vi "Thor_OpenDevice.vi"(8 "error in (no error)":errorcluster) -> (0 "error out":errorcluster, 2 "Device":T2, 3 "KCubeServoControl out":T1, 5 "CreateDevice?":bool)   [LabVIEW 2020]
uses:
  Thor_DeviceRef.ctl
  E:/Norway Project/All Hardware/New Microscope/LabVIEW/ThorLabs/ThorLabs.MotionControl.KCube.DCServoCLI.dll
  ThorLabs.MotionControl.KCube.DCServoCLI.dll
  Thor_KCubeServoDCRef.ctl
  E:/Norway Project/All Hardware/New Microscope/LabVIEW/ThorLabs/Thorlabs.MotionControl.Controls.dll
  Thorlabs.MotionControl.Controls.dll
panel:
  in  "SerialNumber":string="27256317"
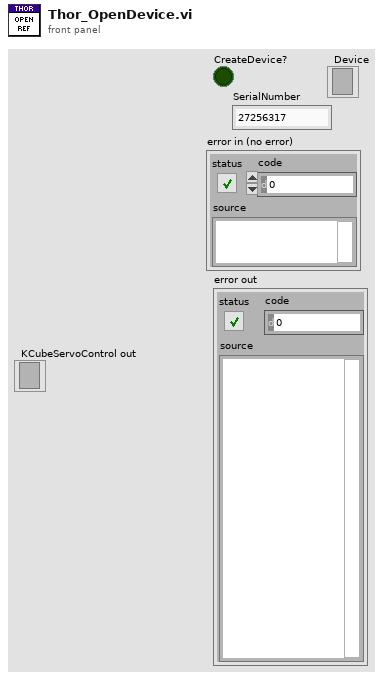
[diagram p1: front panel]
types:
  T1 = typedef "Thor_KCubeServoDCRef.ctl" = refnum<k24>
  T2 = typedef "Thor_DeviceRef.ctl" = refnum<k24>
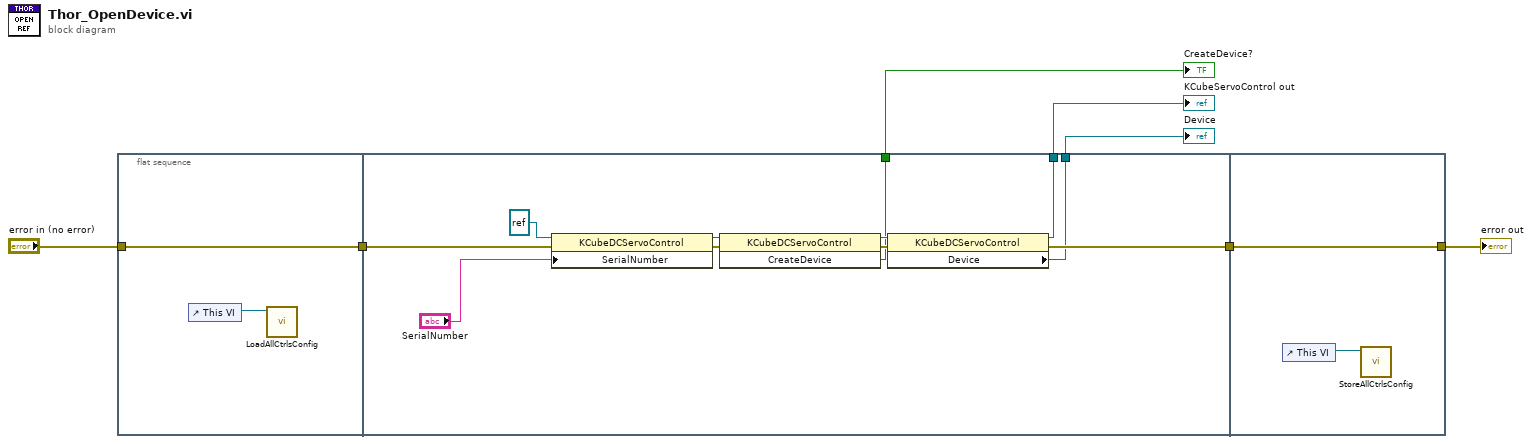
[diagram p0: block diagram]
diagram:
  n1 = flat-sequence {
    tunnel: [w9] -> w6
    tunnel: "error in (no error)" -> [w9]
    tunnel: [w15] -> w7
    tunnel: w6 -> [w14]
    tunnel: [w12] -> w4
    tunnel: [w11] -> w1
    tunnel: [w10] -> w2
    tunnel: w4 -> [w21]
    tunnel: [w21] -> w3
    frame #0 {
      n2 = control-ref of="This VI"() -> (w8:refnum<vi>)
      n3 = call "LoadAllCtrlsConfig.vi"("VI in"=w8) -> ()  [unwired: 11 in]
    }
    frame #1 {
      n4 = property class="KCubeDCServoControl"(reference=refnum<k24> refnum ("KCubeStepperControl In"), error in=w14, "SerialNumber"="SerialNumber") -> (reference out=w17:refnum<k24>, error out=w19:errorcluster)
      n5 = invoke class="KCubeDCServoControl" method="CreateDevice"(reference=w17, error in=w19) -> (reference out=w18:refnum<k24>, error out=w20:errorcluster, "CreateDevice"=w15:bool)  [unwired: 1 in]
      n6 = property class="KCubeDCServoControl"(reference=w18, error in=w20) -> (reference out=w11:refnum<k24>, error out=w12:errorcluster, "Device"=w10:refnum<k24>)
    }
    frame #2 {
      n7 = control-ref of="This VI"() -> (w22:refnum<vi>)
      n8 = call "StoreAllCtrlsConfig.vi"("VI in"=w22) -> ()  [unwired: 11 in]
    }
  }
  "CreateDevice?" <- w7
  "error out" <- w3
  "KCubeServoControl out" <- w1
  "Device" <- w2
